vi "GUI_10TW_MagSpec.vi"() -> ()   [LabVIEW 2013]
uses:
  shared programs/GUI_Template/GUI_master/tcp_new_data_event.ctl
  shared programs/GUI_Template/GUI_master/tcp new data cluster.ctl
  <vilib>/vision/NI_Vision_Development_Module.lvlib
panel:
  in  "Dummy\nCurrent":bool
  out "MagSpec Lineout":cluster{"energy":dbl[], "counts":dbl[]}[](graph)
  in  "confg cluster CamC":T1={"position"=45.72, "field of view"=106.18, "Analysis ROI"=[23, 41, 501, 306]} caption="confg cluster Cam2"
  in  "confg cluster CamB":T1={"position"=142.68, "field of view"=174.3, "Analysis ROI"=[11, 85, 494, 272]}
  in  "confg cluster CamA":T1={"position"=19.22, "field of view"=279.27, "Analysis ROI"=[16, 31, 489, 140]}
  out "image::5":T2(plugin-control) caption="MagSpecC"
  out "MagSpecB":u8[][](graph) caption="MagSpecC"
  out "error out":errorcluster
  out "image::4":T2(plugin-control) caption="MsgSpecB"
  out "MagSpecB":u8[][](graph)
  in  "GUIdevice 5":string="10TW_MagSpecC" caption="MagSpecC"
  in  "GUIdevice 4":string="10TW_MagSpecB" caption="MagSpecB"
  out "MagSpecA":u8[][](graph)
  out "image::3":T2(plugin-control) caption="MagSpecA"
  in  "GUIdevice 3":string="10TW_MagSpecA" caption="MagSpecA"
  out "Status\n% - Ready":dbl(slide) scale=0.0..100.0
  out "AnalogOutput.Channel 0::1":dbl caption="Current Output" min=-10.0 max=10.0
  out "reading.var 5::2":dbl=-0.163229 caption="Current FeedBack" min=-100000.0 max=100000.0
  in  "GUIdevice 2":string="10TW_DAQmultiplier"
  in  "Magnet Current":dbl=-0.163229
  in  "GUIdevice 1":string="10TW_DAQ"
  in  "stop":bool
  out "tcp data event":T3
  out "error IO 2":errorcluster
  # "MAGNET CONTROLS"
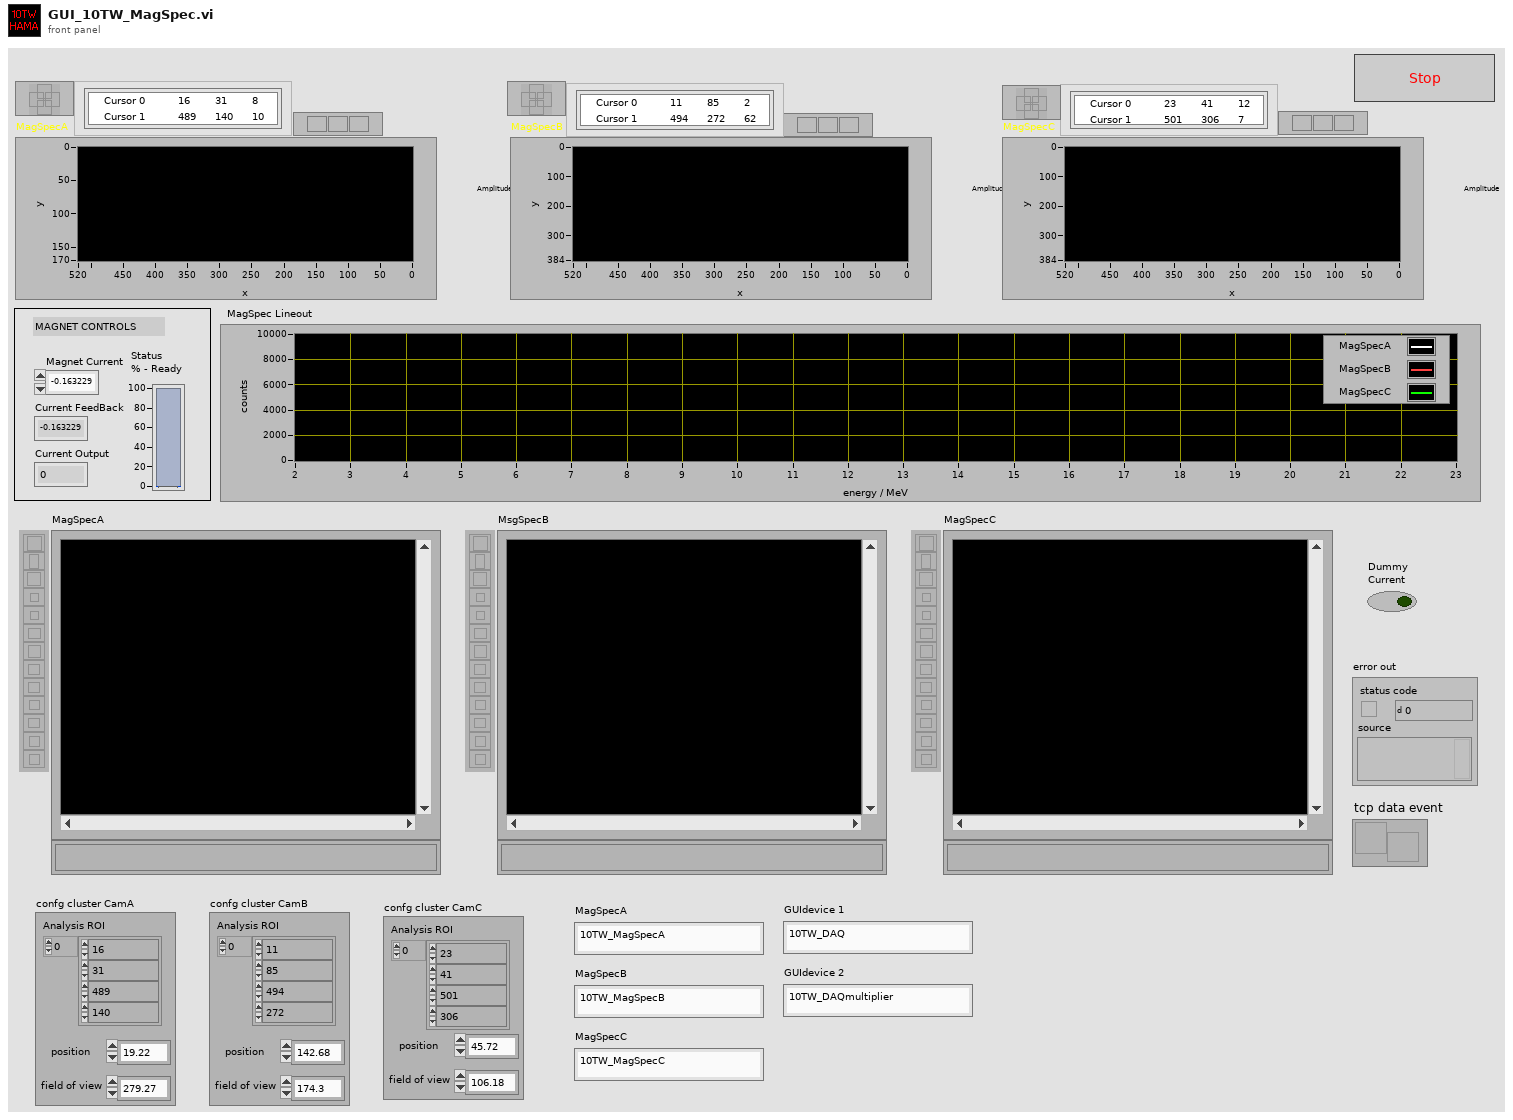
[diagram p1: front panel]
types:
  T1 = cluster{"position":dbl, "field of view":dbl, "Analysis ROI":i32[]}
  T2 = typedef "IMAQ Image.ctl" = refnum<image>
  T3 = typedef "tcp_new_data_event.ctl" = refnum<user-event>
  T4 = typedef "Image Type" = u32
  T5 = typedef "tcp new data cluster.ctl" = cluster{"EventEnum":enum16{"new data", "connection status update"}, "Device name":string}
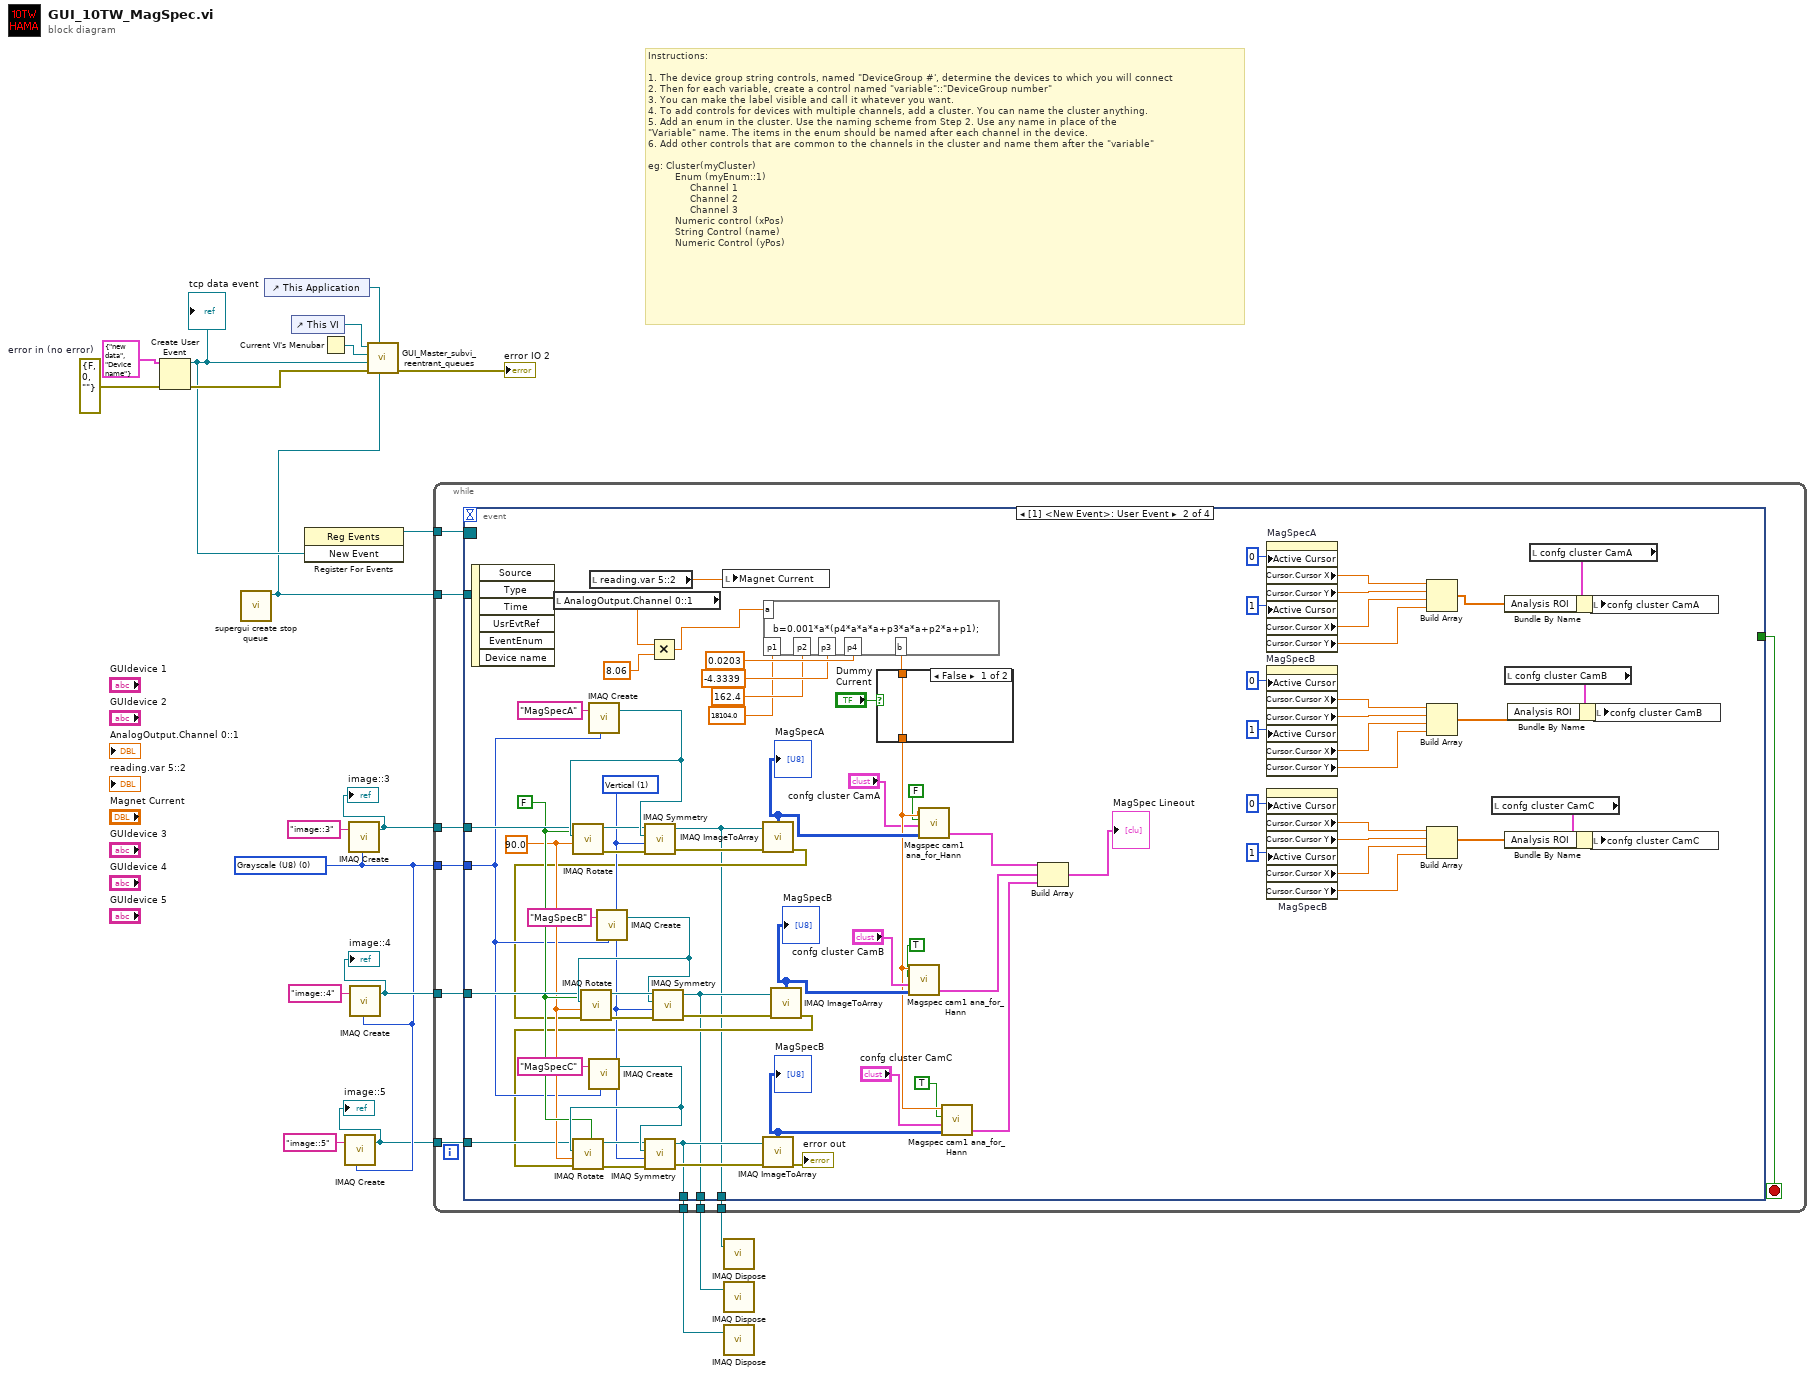
[diagram p0: block diagram]
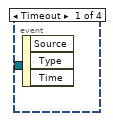
[diagram p2: hidden frame]
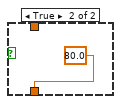
[diagram p3: hidden frame]
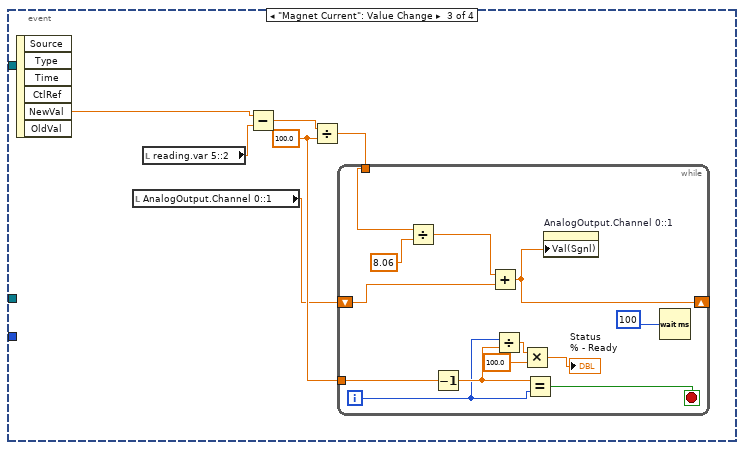
[diagram p4: hidden frame]
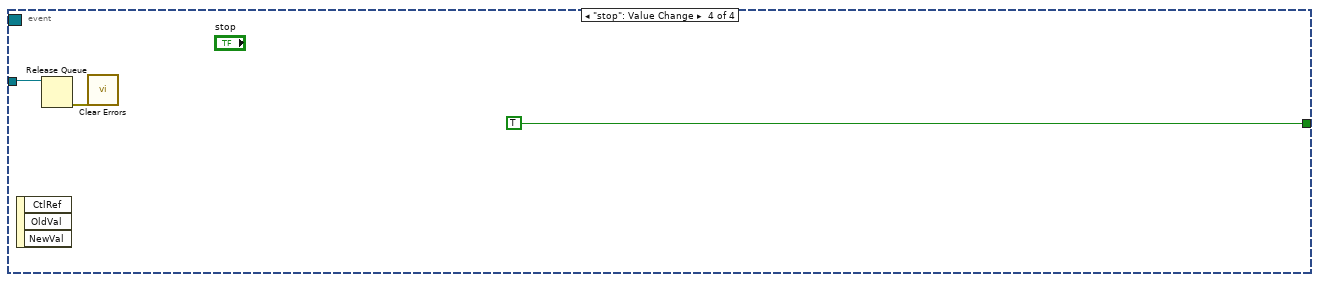
[diagram p5: hidden frame]
diagram:
  w6 = T4 0 items=["Grayscale (U8)", "Grayscale (I16)", "Grayscale (SGL)", "Complex (CSG)", "RGB (U32)", "HSL (U32)", "RGB (U64)", "Grayscale (U16)"] ("Image Type")
  w14 = errorcluster {"status"=FALSE, "code"=0, "source"=""}  # error in (no error)
  # "Instructions:\n\n1. The device group string controls, named \"DeviceGroup #', determine the devices to which you will connect\n2. Then for each variable, create a control named \"variable\"::\"DeviceGroup number\"\n3. You can make the label visible and call it whatever you want.\n4. To add controls for devices with multiple channels, add a cluster. You can name the cluster anything.\n5. Add an enum in the cluster. Use the naming scheme from Step 2. Use any name in place of the \n\"Variable\" name. The items in the enum should be named after each channel in the device. \n6. Add other controls that are common to the channels in the cluster and name them after the \"variable\"\n\neg: Cluster(myCluster)\n         Enum (myEnum::1)\n              Channel 1 \n              Channel 2\n              Channel 3\n         Numeric control (xPos)\n         String Control (name)\n         Numeric Control (yPos)"
  n1 = Create User Event(user event datatype=T5 {"EventEnum"=enum."new data", "Device name"="Device name"} ("New Event"), error in=w14) -> (user event=w13:refnum<user-event>, error out=w16:errorcluster)
  "tcp data event" <- w13
  n2 = call "supergui create stop queue.vi"() -> ("STOP Queue out"=w1:refnum<queue>)  [unwired: 11 in]
  n3 = control-ref of="This Application"() -> (w15:refnum<vi>)
  n4 = control-ref of="This VI"() -> (w19:refnum<vi>)
  n5 = register-events(w13) -> (reference out=w12:refnum<event-registration>)  [unwired: 2 in, 1 out]
  n6 = Current VI's Menubar() -> (w18:refnum<k9>)
  n7 = call "IMAQ Create"("Image Name"="image::5", "Image Type"=w6) -> ("New Image"=w5:T2)  [unwired: 3 in, 1 out]
  "image::5" <- w5
  n8 = call "IMAQ Create"("Image Name"="image::3", "Image Type"=w6) -> ("New Image"=w10:T2)  [unwired: 3 in, 1 out]
  "image::3" <- w10
  n9 = call "IMAQ Create"("Image Name"="image::4", "Image Type"=w6) -> ("New Image"=w8:T2)  [unwired: 3 in, 1 out]
  "image::4" <- w8
  n10 = call "GUI_Master_subvi_reentrant_queues.vi"("STOP Queue in"=w1, "This Application"=w15, "error in (no error)"=w16, "tcp data event"=w13, "Caller menu reference"=w18, "Caller VI ref"=w19) -> ("error out"=→"error IO 2":errorcluster)  [unwired: 5 in]
  n11 = while {
    tunnel: w12 -> [w30]
    tunnel: w10 -> [w28]
    tunnel: w6 -> [w27]
    tunnel: w8 -> [w26]
    tunnel: w5 -> [w25]
    tunnel: [w24] -> w4
    tunnel: [w23] -> w3
    tunnel: [w22] -> w2
    tunnel: w1 -> [w21]
    stop <- w29 stop-if-true
    n12 = event shown="[1] <New Event>: User Event" {
      selector: w30 -> [_ _ _ _]
      dyn-events: _ -> [_ _ _ _]
      timeout: _ -> [_ _ _ _]
      tunnel: [_ _ _ TRUE] -> w29
      tunnel: w28 -> [_ w103 _ _]
      tunnel: w27 -> [_ w87 _ _]
      tunnel: w26 -> [_ w97 _ _]
      tunnel: w25 -> [_ w86 _ _]
      tunnel: [_ w83 _ _] -> w24
      tunnel: [_ w82 _ _] -> w23
      tunnel: [_ w81 _ _] -> w22
      tunnel: w21 -> [_ _ _ w132]
      event Timeout {
        n13 = event-data() -> ()  [unwired: 1 in, 3 out]
      }
      event User Event {
        w90 = u32 1 items=["Horizontal", "Vertical", "Central", "1st Diagonal", "2nd Diagonal"] ("Type of Symmetry")
        w89 = FALSE ("Maintain Size")
        w88 = sgl 90.0 ("Angle (degrees)")
        n14 = event-data() -> ()  [unwired: 1 in, 6 out]
        n15 = local read "AnalogOutput.Channel 0::1"() -> (w71:dbl)
        n16 = call "IMAQ Create"("Image Name"="MagSpecA", "Image Type"=w87) -> ("New Image"=w107:T2)  [unwired: 3 in, 1 out]
        n17 = call "IMAQ Rotate"("Maintain Size"=w89, "Angle (degrees)"=w88, "Image Dst"=w107, "Image Src"=w103) -> ("error out"=w105:errorcluster, "Image Dst Out"=w104:T2)  [unwired: 4 in, 2 out]
        n18 = call "IMAQ Create"("Image Name"="MagSpecC", "Image Type"=w87) -> ("New Image"=w94:T2)  [unwired: 3 in, 1 out]
        n19 = local read "reading.var 5::2"() -> (w109:dbl)
        n20 = call "IMAQ Create"("Image Name"="MagSpecB", "Image Type"=w87) -> ("New Image"=w99:T2)  [unwired: 3 in, 1 out]
        n21 = call "IMAQ Symmetry"("error in (no error)"=w105, "Type of Symmetry"=w90, "Image Dst"=w107, "Image Src"=w104) -> ("error out"=w108:errorcluster, "Image Dst Out"=w81:T2)  [unwired: 1 out]
        n22 = Multiply(x=w71, y=8.06) -> (x*y=w69:dbl)
        n23 = local write "Magnet Current"(w109) -> ()
        n24 = call "IMAQ ImageToArray"("error in (no error)"=w108, "Image"=w81) -> ("error out"=w85:errorcluster, "Image Pixels (U8)"=w76:u8[][])  [unwired: 1 in, 4 out]
        "MagSpecA" <- w76
        n25 = call "IMAQ Rotate"("Maintain Size"=w89, "error in (no error)"=w85, "Angle (degrees)"=w88, "Image Dst"=w99, "Image Src"=w97) -> ("error out"=w101:errorcluster, "Image Dst Out"=w102:T2)  [unwired: 3 in, 2 out]
        n26 = call "IMAQ Symmetry"("error in (no error)"=w101, "Type of Symmetry"=w90, "Image Dst"=w99, "Image Src"=w102) -> ("error out"=w98:errorcluster, "Image Dst Out"=w82:T2)  [unwired: 1 out]
        n27 = formula code="b=0.001*a*(p4*a*a*a+p3*a*a+p2*a+p1);"("a"=w69, "p4"=0.0203 ("input variable"), "p3"=-4.3339 ("input variable"), "p2"=162.4 ("input variable"), "p1"=18104.0 ("input variable")) -> ("b"=w32:dbl)
        n28 = call "IMAQ ImageToArray"("error in (no error)"=w98, "Image"=w82) -> ("error out"=w84:errorcluster, "Image Pixels (U8)"=w79:u8[][])  [unwired: 1 in, 4 out]
        "MagSpecB" <- w79
        n29 = call "IMAQ Rotate"("Maintain Size"=w89, "error in (no error)"=w84, "Angle (degrees)"=w88, "Image Dst"=w94, "Image Src"=w86) -> ("error out"=w92:errorcluster, "Image Dst Out"=w91:T2)  [unwired: 3 in, 2 out]
        n30 = call "IMAQ Symmetry"("error in (no error)"=w92, "Type of Symmetry"=w90, "Image Dst"=w94, "Image Src"=w91) -> ("error out"=w95:errorcluster, "Image Dst Out"=w83:T2)  [unwired: 1 out]
        n31 = call "IMAQ ImageToArray"("error in (no error)"=w95, "Image"=w83) -> ("error out"=→"error out":errorcluster, "Image Pixels (U8)"=w78:u8[][])  [unwired: 1 in, 4 out]
        "MagSpecB" <- w78
        n32 = case shown="False" "Dummy\nCurrent" {
          tunnel: [w110 80.0 ("B [mT]")] -> w68
          tunnel: w32 -> [w110 _]
          frame False {
          }
          frame True {
          }
        }
        n33 = call "Magspec cam1 ana_for_Hann.vi"("Image I16"=w79, "confg cluster"="confg cluster CamB", "true4Fwd"=TRUE, "B [mT]"=w68) -> ("XY Graph"=w66:cluster{"energy":dbl[], "counts":dbl[]})  [unwired: 2 out]
        n34 = call "Magspec cam1 ana_for_Hann.vi"("Image I16"=w76, "confg cluster"="confg cluster CamA", "true4Fwd"=FALSE, "B [mT]"=w68) -> ("XY Graph"=w67:cluster{"energy":dbl[], "counts":dbl[]})  [unwired: 2 out]
        n35 = call "Magspec cam1 ana_for_Hann.vi"("Image I16"=w78, "confg cluster"="confg cluster CamC", "true4Fwd"=TRUE, "B [mT]"=w68) -> ("XY Graph"=w64:cluster{"energy":dbl[], "counts":dbl[]})  [unwired: 2 out]
        n36 = Build Array(w67, w66, w64) -> (→"MagSpec Lineout":cluster{"energy":dbl[], "counts":dbl[]}[])
        n37 = property on="MagSpecA" class="IntGraph (strict)"("Active Cursor"=u32 0, "Active Cursor"=u32 1) -> ("Cursor.Cursor X"=w61:dbl, "Cursor.Cursor Y"=w62:dbl, "Cursor.Cursor X"=w63:dbl, "Cursor.Cursor Y"=w58:dbl)  [unwired: 2 in, 2 out]
        n38 = property on="MagSpecB" class="IntGraph (strict)"("Active Cursor"=u32 0, "Active Cursor"=u32 1) -> ("Cursor.Cursor X"=w54:dbl, "Cursor.Cursor Y"=w53:dbl, "Cursor.Cursor X"=w52:dbl, "Cursor.Cursor Y"=w57:dbl)  [unwired: 2 in, 2 out]
        n39 = property on="MagSpecB" class="IntGraph (strict)"("Active Cursor"=u32 0, "Active Cursor"=u32 1) -> ("Cursor.Cursor X"=w49:dbl, "Cursor.Cursor Y"=w50:dbl, "Cursor.Cursor X"=w51:dbl, "Cursor.Cursor Y"=w46:dbl)  [unwired: 2 in, 2 out]
        n40 = Build Array(w61, w62, w63, w58) -> (w44:dbl[])
        n41 = Build Array(w54, w53, w52, w57) -> (w39:dbl[])
        n42 = Build Array(w49, w50, w51, w46) -> (w37:dbl[])
        n43 = local read "confg cluster CamC"() -> (w38:T1)
        n44 = local read "confg cluster CamB"() -> (w41:T1)
        n45 = Bundle By Name(cluster=w38, "Analysis ROI"=w37) -> (w36:T1)
        n46 = Bundle By Name(cluster=w41, "Analysis ROI"=w39) -> (w40:T1)
        n47 = local read "confg cluster CamA"() -> (w43:T1)
        n48 = Bundle By Name(cluster=w43, "Analysis ROI"=w44) -> (w42:T1)
        n49 = local write "confg cluster CamA"(w42) -> ()
        n50 = local write "confg cluster CamC"(w36) -> ()
        n51 = local write "confg cluster CamB"(w40) -> ()
      }
      event "Magnet Current": Value Change {
        w116 = 100.0 ("y")
        n52 = event-data() -> ("NewVal"=w113:dbl)  [unwired: 1 in, 5 out]
        n53 = local read "AnalogOutput.Channel 0::1"() -> (w112:dbl)
        n54 = local read "reading.var 5::2"() -> (w117:dbl)
        n55 = Subtract(x=w113, y=w117) -> (x-y=w115:dbl)
        n56 = Divide(x=w115, y=w116) -> (x/y=w114:dbl)
        n57 = while {
          tunnel: w116 -> [w128]
          tunnel: w114 -> [w122]
          shift-right: [w118] -> _
          shift-left: w112 -> [w119]
          i -> [w126]
          stop <- w130 stop-if-true
          n58 = Divide(x=w122, y=8.06) -> (x/y=w121:dbl)
          n59 = Decrement(x=w128) -> (x-1=w127:dbl)
          n60 = Add(x=w121, y=w119) -> (x+y=w118:dbl)
          n61 = Divide(x=w126, y=w127) -> (x/y=w125:dbl)
          n62 = Multiply(x=w125, y=100.0) -> (x*y=→"Status\n% - Ready":dbl)
          n63 = Equal?(x=w127, y=w126) -> (x = y?=w130:bool)
          n64 = property on="AnalogOutput.Channel 0::1" class="DigNum (strict)"("Val(Sgnl)"=w118) -> ()  [unwired: 2 in, 2 out]
          n65 = Wait (ms)(milliseconds to wait=u32 100) -> ()  [unwired: 1 out]
        }
      }
      event "stop": Value Change {
        n66 = event-data() -> ()  [unwired: 1 in, 3 out]
        n67 = Release Queue(queue=w132) -> (error out=w131:errorcluster)  [unwired: 2 in, 2 out]
        n68 = call <vilib>:"Clear Errors.vi"("error in (no error)"=w131) -> ()  [unwired: 6 in, 1 out]
      }
    }
  }
  n69 = call "IMAQ Dispose"("Image"=w2) -> ()  [unwired: 5 in, 1 out]
  n70 = call "IMAQ Dispose"("Image"=w3) -> ()  [unwired: 5 in, 1 out]
  n71 = call "IMAQ Dispose"("Image"=w4) -> ()  [unwired: 5 in, 1 out]
